vi "PH_Cont-601k_PSU.Test.vi"() -> ()   [LabVIEW 2014, in "PH_Cont-601k_PSU.lvlib"]
uses:
  PH_Cont-601k_PSU.lvlib
  PH_Cont-601k_PSU.Device Status.ctl
  PH_Cont-601k_PSU.Mode.ctl
  instr.lib/pu601k/Public/Action-Status/LaserStatus.ctl
  instr.lib/pu601k/Public/Action-Status/InterlockStatus.ctl
  PH_Basics/PH_Common/PH_Common.lvlib
  instr.lib/pu601k/Continuum PU610K.lvlib
panel:
  in  "LaserStatus":T1 {"Laser State" items=["STOP: Stop Mode"=0, "STOP: Retrieve laser head serial number"=2, "STOP: Read flash and Q-switch counters"=3, "STOP: Keyswitch off"=5, "STOP: Delay for SmartBoard to get ready"=4, "STOP: SmartBoard download initialization"=6, "STOP: Retrieve SmartBoard version information"=7, "STOP: Retrieve all infos from SmartBoard"=8, "STOP: Stop Initialization"=10, "STOP: At Power-ON, found RUN, waiting for STOP"=15, "STOP: Idle, waiting for commands"=20, "STOP: Init laser head downloading process"=25, "STOP: Retrieve SmartBoard EEPROM location"=27, "STOP: Download laser head data"=30, "STOP: Initialize Power On Self Tests"=35, "STOP: Power On Self Test: Wait for pump to turn on"=40, "STOP: Power On Self Test: Wait for shutter to close"=45, "STOP: Power On Self Test: Wait for shutter to open"=50, "STANDBY: Standby Mode"=100, "STANDBY: Standby Initialization"=110, "STANDBY: Waiting for SmartBoard to complete a task"=113, "STANDBY: Idle, waiting for commands"=120, "STANDBY: Waiting for Smart Board to complete a task"=123, "STANDBY: At Power-ON, found READY. Waiting for STANDBY"=130, "READY: Ready Mode"=200, "READY: Ready Mode Initialization"=205, "READY: Begin Charging"=206, "READY: Wait for initial capacitor charge"=207, "READ: Charging???"=208, "READY: Initial charge completion"=209, "READY: Idle, waiting for commands"=210, "READY: Uploading of paramters to the laser head"=215, "EMISSION: Emission Mode"=300, "EMISSION: Idle, waiting for commands"=310, "EMISSION: Waiting for shutter to close"=311, "EMISSION: Waiting to set pyro"=313, "EMISSION: Servo control to hold value"=315, "EMISSION: Servo context monitoring"=320, "EMISSION: Initialization for laser head pyro gein adjustment"=330, "EMISSION: Pyro gain adjustment - step 1"=335, "EMISSION: Pyro gain adjustment - step 2"=340, "EMISSION: Pyro gain adjustment - step 3"=345, "EMISSION: Pyro gain adjustment complete"=350, "ERROR: Error Mode"=400, "ERROR: Initialization for error mode"=405, "ERROR: Cooling Error - wating for STOP"=410, "ERROR: Error control for laser head not initialized fault."=415, "ERROR: Error control for TS-485 (Smart Bus) fault."=420, "ERROR: Error control for cover interlocks"=425, "ERROR: Watchdog timeout"=435]}
  out "Configuration change is allowed":bool
  out "Charge is allowed":bool
  out "Mode":T3
  in  "error message":string
  in  "EOC reached?":bool
  out "output cluster":T4={"State"=0, "Interlocks"=[], "EOC"=16860, "Flashlamp Counter"=0, "error message"=""} {"State" items=["STOP: Stop Mode"=0, "STOP: Retrieve laser head serial number"=2, "STOP: Read flash and Q-switch counters"=3, "STOP: Keyswitch off"=5, "STOP: Delay for SmartBoard to get ready"=4, "STOP: SmartBoard download initialization"=6, "STOP: Retrieve SmartBoard version information"=7, "STOP: Retrieve all infos from SmartBoard"=8, "STOP: Stop Initialization"=10, "STOP: At Power-ON, found RUN, waiting for STOP"=15, "STOP: Idle, waiting for commands"=20, "STOP: Init laser head downloading process"=25, "STOP: Retrieve SmartBoard EEPROM location"=27, "STOP: Download laser head data"=30, "STOP: Initialize Power On Self Tests"=35, "STOP: Power On Self Test: Wait for pump to turn on"=40, "STOP: Power On Self Test: Wait for shutter to close"=45, "STOP: Power On Self Test: Wait for shutter to open"=50, "STANDBY: Standby Mode"=100, "STANDBY: Standby Initialization"=110, "STANDBY: Waiting for SmartBoard to complete a task"=113, "STANDBY: Idle, waiting for commands"=120, "STANDBY: Waiting for Smart Board to complete a task"=123, "STANDBY: At Power-ON, found READY. Waiting for STANDBY"=130, "READY: Ready Mode"=200, "READY: Ready Mode Initialization"=205, "READY: Begin Charging"=206, "READY: Wait for initial capacitor charge"=207, "READY: Charging"=208, "READY: Initial charge completion"=209, "READY: Idle, waiting for commands"=210, "READY: Uploading of paramters to the laser head"=215, "EMISSION: Emission Mode"=300, "EMISSION: Idle, waiting for commands"=310, "EMISSION: Waiting for shutter to close"=311, "EMISSION: Waiting to set pyro"=313, "EMISSION: Servo control to hold value"=315, "EMISSION: Servo context monitoring"=320, "EMISSION: Initialization for laser head pyro gein adjustment"=330, "EMISSION: Pyro gain adjustment - step 1"=335, "EMISSION: Pyro gain adjustment - step 2"=340, "EMISSION: Pyro gain adjustment - step 3"=345, "EMISSION: Pyro gain adjustment complete"=350, "ERROR: Error Mode"=400, "ERROR: Initialization for error mode"=405, "ERROR: Cooling Error - wating for STOP"=410, "ERROR: Error control for laser head not initialized fault."=415, "ERROR: Error control for TS-485 (Smart Bus) fault."=420, "ERROR: Error control for cover interlocks"=425, "ERROR: Watchdog Timeout"=435]}
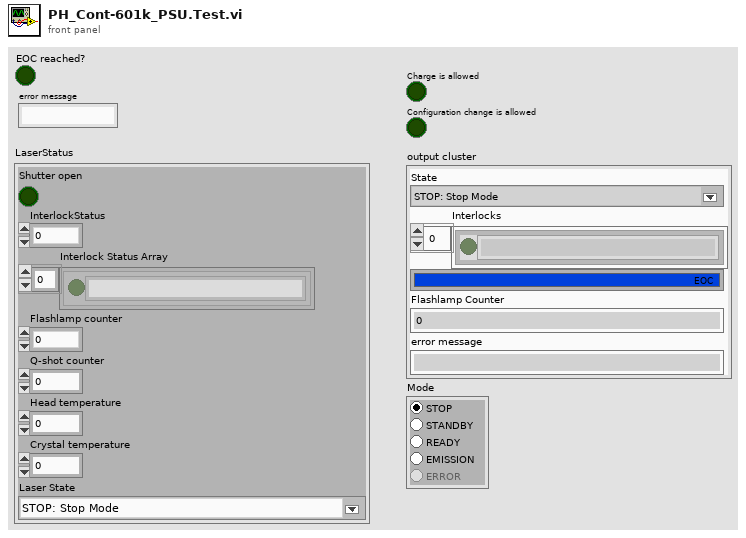
[diagram p1: front panel]
types:
  T1 = typedef "Continuum PU610K.lvlib/LaserStatus.ctl" = cluster{"Shutter open":bool, "InterlockStatus":u16, "Interlock Status Array":T2[], "Flashlamp counter":u32, "Q-shot counter":u32, "Head temperature":u16, "Crystal temperature":u16, "Laser State":u16}
  T2 = typedef "Continuum PU610K.lvlib/InterlockStatus.ctl" = cluster{"on/off":bool, "Explanation":string}
  T3 = typedef "PH_Cont-601k_PSU.lvlib/PH_Cont-601k_PSU.Mode.ctl" = enum32{"STOP", "STANDBY", "READY", "EMISSION", "ERROR"}
  T4 = typedef "PH_Cont-601k_PSU.lvlib/PH_Cont-601k_PSU.Device Status.ctl" = cluster{"State":u16, "Interlocks":cluster{"on/off":bool, "Explanation":string}[], "EOC":u32, "Flashlamp Counter":u32, "error message":string}
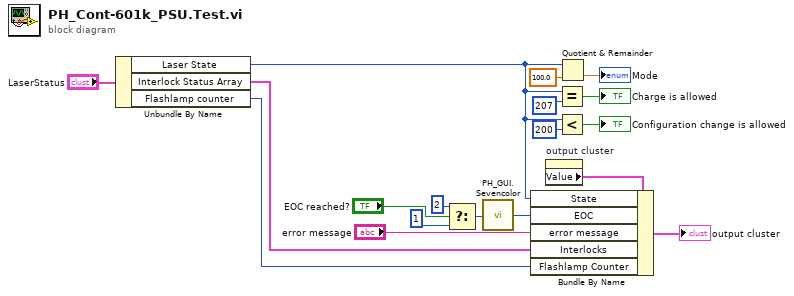
[diagram p0: block diagram]
diagram:
  n1 = Unbundle By Name("LaserStatus") -> ("Laser State"=w1:u16, "Interlock Status Array"=w3:T2[], "Flashlamp counter"=w2:u32)
  n2 = Select(t=2 ("EOC"), s="EOC reached?", f=1 ("EOC")) -> (s? t:f=w6:i32)
  n3 = call "PH_GUI.Sevencolor.vi"("State"=w6) -> ("Color Box"=w5:u32)
  n4 = property on="output cluster" class="Clust (strict)"() -> ("Value"=w13:T4)  [unwired: 2 in, 2 out]
  n5 = Bundle By Name(cluster=w13, "State"=w1, "EOC"=w5, "error message"="error message", "Interlocks"=w3, "Flashlamp Counter"=w2) -> (→"output cluster":T4)
  n6 = Equal?(x=w1, y=u16 207) -> (x = y?=→"Charge is allowed":bool)
  n7 = Less?(x=w1, y=u16 200) -> (x < y?=→"Configuration change is allowed":bool)
  n8 = Quotient & Remainder(x=w1, y=100.0) -> (floor(x/y)=→"Mode":dbl)  [unwired: 1 out]
